vi "Header String (String).vi"(10 "Value":string, 11 "Name":string) -> (3 "Header":string)   [LabVIEW 2020, in "HTTP Utils.lvlib"]
uses:
  HTTP Utils.lvlib
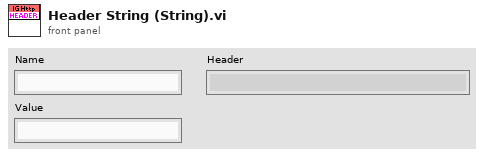
[diagram p1: front panel]
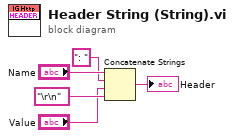
[diagram p0: block diagram]
diagram:
  n1 = Concatenate Strings("Name", ": " ("string"), "Value", "\r\n" ("string")) -> (→"Header":string)
